vi "Get index from key(decimal).vi"(8 "error in (no error)":errorcluster, 9 "Value(decimal)":u64, 10 "key":string, 11 "VElement":variant) -> (0 "error out":errorcluster, 3 "indexOut":i32)   [LabVIEW 2015]
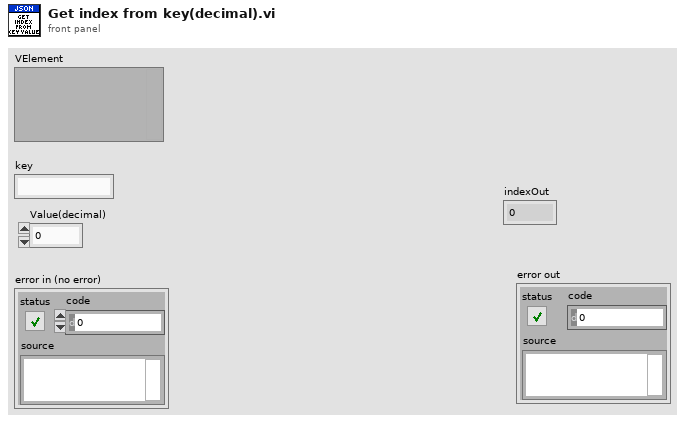
[diagram p1: front panel]
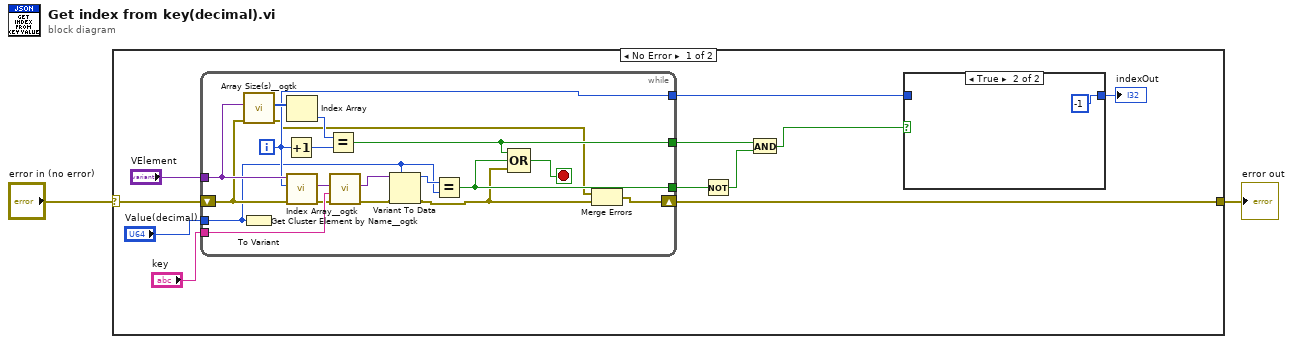
[diagram p0: block diagram]
diagram:
  n1 = case shown="No Error" "error in (no error)" {
    selector: "error in (no error)" -> [w12 w35]
    tunnel: [w10 w35] -> w1
    frame No Error {
      n2 = while {
        tunnel: "VElement" -> [w31]
        tunnel: "key" -> [w33]
        tunnel: "Value(decimal)" -> [w16]
        tunnel: [w29] -> w5
        shift-right: [w21] -> w10
        shift-left: w12 -> [w23]
        tunnel: [w25] -> w8
        tunnel: [w26] -> w9
        i -> [w29]
        stop <- w24 stop-if-true
        n3 = call <userlib>:"Array Size(s)__ogtk.vi"("error in (no error)"=w23, "Array"=w31) -> ("error out"=w22:errorcluster, "Size(s)"=w30:u32[])  [unwired: 7 in, 1 out]
        n4 = To Variant(anything=w16) -> ()  [unwired: 1 out]
        n5 = Increment(x=w29) -> (x+1=w27:i32)
        n6 = Index Array(array=w30) -> (element=w28:u32)  [unwired: 1 in]
        n7 = call <userlib>:"Index Array__ogtk.vi"("error in (no error)"=w23, "Index (1D)"=w29, "MultiD Array"=w31) -> ("error out"=w32:errorcluster, "Array Element"=w34:variant)  [unwired: 7 in]
        n8 = Equal?(x=w28, y=w27) -> (x = y?=w25:bool)
        n9 = call <userlib>:"Get Cluster Element by Name__ogtk.vi"("error in (no error)"=w32, "Element Name"=w33, "Cluster"=w34) -> ("error out"=w20:errorcluster, "VElement"=w18:variant)  [unwired: 6 in, 1 out]
        n10 = Variant To Data(error in=w20, type=w16, Variant=w18) -> (data=w17:u64, error out=w19:errorcluster)
        n11 = Equal?(x=w17, y=w16) -> (x = y?=w26:bool)
        n12 = Compound Arithmetic op=OR(w25, w26, w19) -> (w24:bool)
        n13 = Merge Errors(w22, w19) -> (w21:errorcluster)
      }
      n14 = Not(x=w9) -> (.not. x?=w7:bool)
      n15 = And(x=w8, y=w7) -> (x .and. y?=w4:bool)
      n16 = case shown="True" w4 {
        tunnel: w5 -> [w14 _]
        tunnel: [w14 -1] -> w3
        frame False {
        }
        frame True {
        }
      }
      "indexOut" <- w3
    }
    frame Error {
    }
  }
  "error out" <- w1
